vi "IdleCheck.vi"(8 "error in (no error)":errorcluster, 11 "S2.lvclass":refnum<class "S5.lvclass">) -> (0 "error out":errorcluster)   [LabVIEW 2018, in "S5.lvclass"]
uses:
  S5.lvclass
  S5.lvclass/S5.ctl
  GUI3/GUI3.lvclass
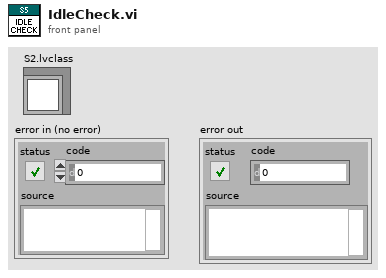
[diagram p1: front panel]
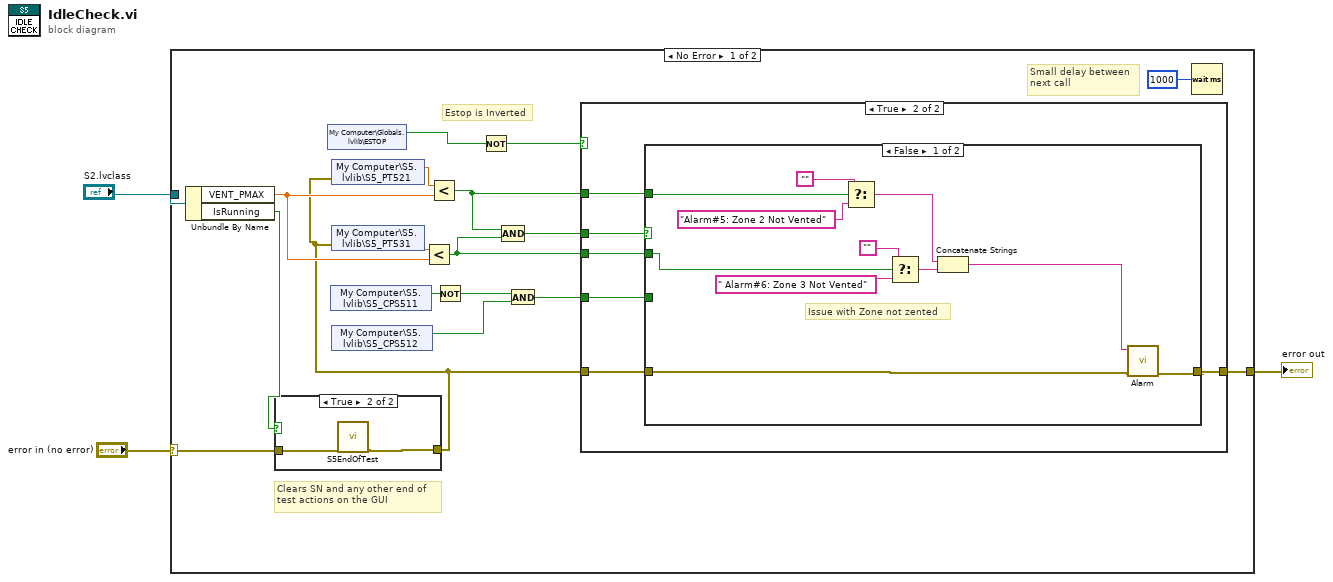
[diagram p0: block diagram]
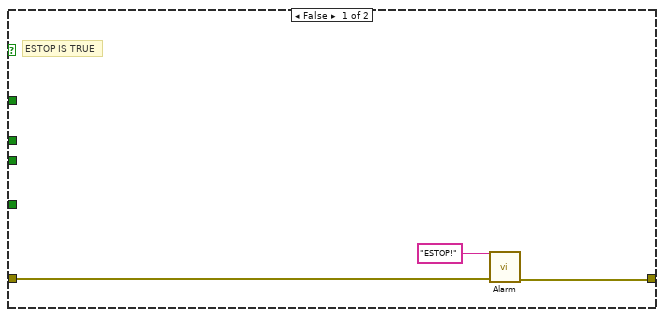
[diagram p3: hidden frame]
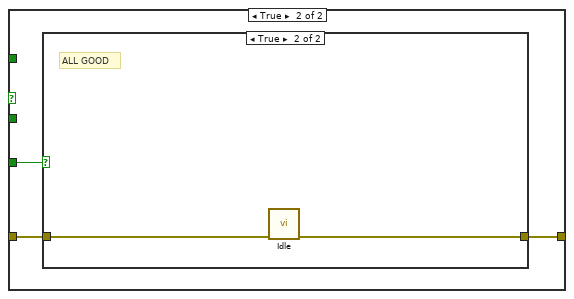
[diagram p4: hidden frame]
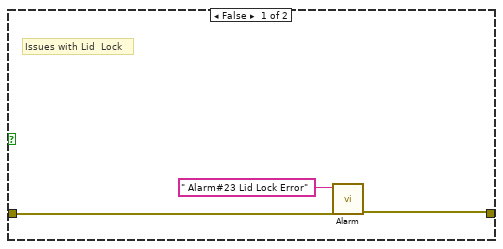
[diagram p5: hidden frame]
diagram:
  n1 = case shown="No Error" "error in (no error)" {
    selector: "error in (no error)" -> [w5 w53]
    tunnel: [w18 w53] -> w2
    tunnel: "S2.lvclass" -> [w8 _]
    frame No Error {
      # "Clears SN and any other end of\ntest actions on the GUI"
      # "Small delay between\nnext call"
      # "Estop is Inverted"
      n2 = Unbundle By Name(w8) -> ("VENT_PMAX"=w7:dbl, "IsRunning"=w6:bool)
      n3 = case shown="True" w6 {
        tunnel: w5 -> [w22 w24]
        tunnel: [w22 w23] -> w4
        frame False {
        }
        frame True {
          n4 = call "S5EndOfTest.vi"("error in"=w24) -> ("error out"=w23:errorcluster)  [unwired: 10 in]
        }
      }
      n5 = shared-variable "My Computer\\Globals.lvlib\\ESTOP"() -> (w11:bool)  [unwired: 1 in, 1 out]
      n6 = shared-variable "My Computer\\S5.lvlib\\S5_CPS511"() -> (w15:bool)  [unwired: 1 in, 1 out]
      n7 = shared-variable "My Computer\\S5.lvlib\\S5_PT521"(error in=w4) -> (w21:dbl)  [unwired: 1 out]
      n8 = shared-variable "My Computer\\S5.lvlib\\S5_PT531"(error in=w4) -> (w20:dbl)  [unwired: 1 out]
      n9 = shared-variable "My Computer\\S5.lvlib\\S5_CPS512"() -> (w14:bool)  [unwired: 1 in, 1 out]
      n10 = Less?(x=w20, y=w7) -> (x < y?=w16:bool)
      n11 = Less?(x=w21, y=w7) -> (x < y?=w17:bool)
      n12 = Not(x=w15) -> (.not. x?=w10:bool)
      n13 = Not(x=w11) -> (.not. x?=w9:bool)
      n14 = Compound Arithmetic op=AND(w17, w16) -> (w19:bool)
      n15 = And(x=w10, y=w14) -> (x .and. y?=w13:bool)
      n16 = case shown="True" w9 {
        tunnel: w19 -> [_ w33]
        tunnel: [w26 w32] -> w18
        tunnel: w17 -> [_ w31]
        tunnel: w16 -> [_ w30]
        tunnel: w4 -> [w27 w29]
        tunnel: w13 -> [_ w28]
        frame False {
          # "ESTOP IS TRUE"
          n17 = call "Alarm.vi"("error in"=w27, "Alarm"="ESTOP!" ("f")) -> ("error out"=w26:errorcluster)  [unwired: 9 in]
        }
        frame True {
          n18 = case shown="False" w33 {
            tunnel: w29 -> [w34 w47]
            tunnel: [w36 w46] -> w32
            tunnel: w31 -> [w44 _]
            tunnel: w30 -> [w39 _]
            tunnel: w28 -> [_ w45]
            frame False {
              # "Issue with Zone not zented"
              n19 = Select(t="", s=w44, f="Alarm#5: Zone 2 Not Vented" ("Status")) -> (s? t:f=w38:string)
              n20 = Select(t="", s=w39, f=" Alarm#6: Zone 3 Not Vented" ("Status")) -> (s? t:f=w37:string)
              n21 = Concatenate Strings(w38, w37) -> (w35:string)
              n22 = call "Alarm.vi"("error in"=w34, "Alarm"=w35) -> ("error out"=w36:errorcluster)  [unwired: 9 in]
            }
            frame True {
              n23 = case shown="True" w45 {
                tunnel: w47 -> [w50 w52]
                tunnel: [w49 w51] -> w46
                frame False {
                  # "Issues with Lid  Lock"
                  n24 = call "Alarm.vi"("error in"=w50, "Alarm"=" Alarm#23 Lid Lock Error" ("Status")) -> ("error out"=w49:errorcluster)  [unwired: 9 in]
                }
                frame True {
                  # "ALL GOOD"
                  n25 = call "Idle.vi"("error in"=w52) -> ("error out"=w51:errorcluster)  [unwired: 10 in]
                }
              }
            }
          }
        }
      }
      n26 = Wait (ms)(milliseconds to wait=u32 1000) -> ()  [unwired: 1 out]
    }
    frame Error {
    }
  }
  "error out" <- w2
